vi "Untitled 6.vi"() -> ()   [LabVIEW 2011]
panel:
  in  "Numeric":sgl
  out "x << y":u32 format="%b"
  out "x rotated left by y":i16 format="%b"
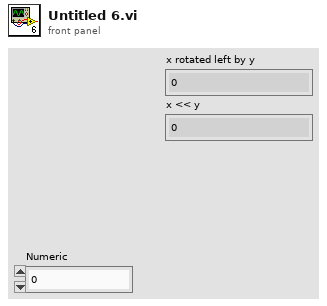
[diagram p1: front panel]
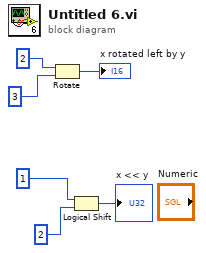
[diagram p0: block diagram]
diagram:
  n1 = Rotate(1:i16 3 ("x"), 2:i16 2 ("y")) -> (0:→"x rotated left by y":i16)
  n2 = Logical Shift(y=i8 1, x=u32 2) -> (x << y=→"x << y":u32)
